vi "Save PNG File.vi"() -> (0 "ErrOut":errorcluster)   [LabVIEW 2017]
doc: "Use this template to build a VI to use as a subVI."
panel:
  out "ImageOut":T1(plugin-control)
  in  "ErrIn":errorcluster
  # "Input Parameters"
  # "Output Parameters"
  # "VI Description:\nThis VI is .."
  # ":: MVI Framework V1.0 ::\nAuthor:Gaoke Yang\nEmail: gaoke.yang@yahoo.com\nWeb: www.mvicontrol.com\nCopyright (C) , MVI Technologies All Rights Reserved"
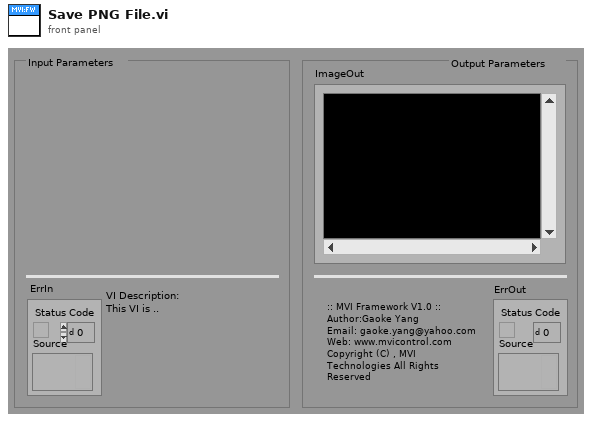
[diagram p1: front panel]
types:
  T1 = typedef "IMAQ Image.ctl" = refnum<image>
  T2 = typedef "Image Type" = u32
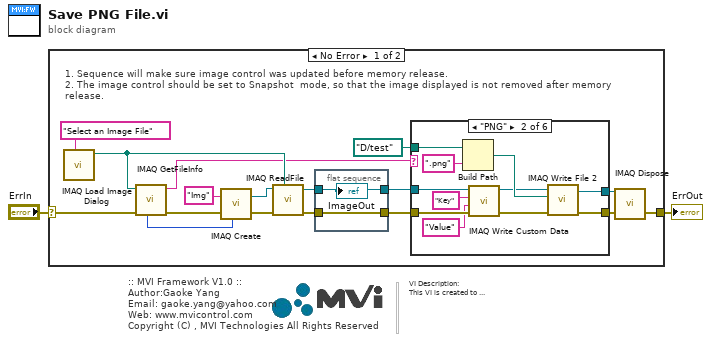
[diagram p0: block diagram]
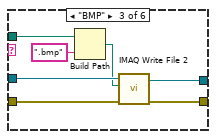
[diagram p3: hidden frame]
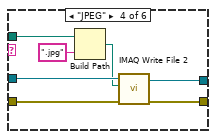
[diagram p4: hidden frame]
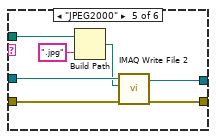
[diagram p5: hidden frame]
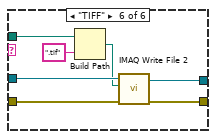
[diagram p6: hidden frame]
diagram:
  # "VI Description:\nThis VI is created to ..."
  # ":: MVI Framework V1.0 ::\nAuthor:Gaoke Yang\nEmail: gaoke.yang@yahoo.com\nWeb: www.mvicontrol.com\nCopyright (C) , MVI Technologies All Rights Reserved"
  n1 = case shown="No Error" "ErrIn" {
    selector: "ErrIn" -> [w14 w62]
    tunnel: [w13 w62] -> w2
    frame No Error {
      # "1. Sequence will make sure image control was updated before memory release.\n2. The image control should be set to Snapshot  mode, so that the image displayed is not removed after memory release."
      n2 = call "IMAQ Load Image Dialog"("Prompt"="Select an Image File" ("prompt")) -> ("Path"=w11:path)  [unwired: 8 in, 2 out]
      n3 = call "IMAQ GetFileInfo"("error in (no error)"=w14, "File Path"=w11) -> ("error out"=w15:errorcluster, "File Type"=w4:string, "Image Type"=w5:T2)  [unwired: 3 in, 4 out]
      n4 = call "IMAQ Create"("Image Name"="Img", "Image Type"=w5, "error in (no error)"=w15) -> ("New Image"=w18:T1, "error out"=w17:errorcluster)  [unwired: 2 in]
      n5 = call "IMAQ ReadFile"("File Path"=w11, "error in (no error)"=w17, "Image"=w18) -> ("error out"=w12:errorcluster, "Image Out"=w10:T1)  [unwired: 4 in, 3 out]
      n6 = flat-sequence {
        tunnel: w10 -> [w60]
        tunnel: w12 -> [w61]
        tunnel: [w61] -> w8
        tunnel: [w60] -> w3
        frame #0 {
          "ImageOut" <- w60
        }
      }
      n7 = case shown="\"PNG\"" w4 {
        tunnel: w3 -> [w21 w31 w38 w45 w52 w59]
        tunnel: [w21 w29 w36 w43 w50 w57] -> w9
        tunnel: w8 -> [w20 w30 w37 w44 w51 w58]
        tunnel: [w20 w28 w35 w42 w49 w56] -> w7
        tunnel: path "D:/test" ("File Path") -> [_ w26 w33 w40 w47 w54]
        frame "xxx", Default {
          # "unkown file type, do nothing"
        }
        frame "PNG" {
          n8 = Build Path(base path=w26, name or relative path=".png") -> (appended path=w27:path)
          n9 = call "IMAQ Write Custom Data"("Custom Data In"="Value", "Key"="Key", "Image"=w31) -> ("Image Out"=w24:T1)  [unwired: 7 in, 1 out]
          n10 = call-poly "IMAQ Write File 2"("error in (no error)"=w30, "File Path"=w27, "Image"=w24) -> ("error out"=w28:errorcluster, "Image Out (duplicate)"=w29:T1)  [unwired: 7 in]
        }
        frame "BMP" {
          n11 = Build Path(base path=w33, name or relative path=".bmp") -> (appended path=w34:path)
          n12 = call-poly "IMAQ Write File 2"("error in (no error)"=w37, "File Path"=w34, "Image"=w38) -> ("error out"=w35:errorcluster, "Image Out (duplicate)"=w36:T1)  [unwired: 7 in]
        }
        frame "JPEG" {
          n13 = Build Path(base path=w40, name or relative path=".jpg") -> (appended path=w41:path)
          n14 = call-poly "IMAQ Write File 2"("error in (no error)"=w44, "File Path"=w41, "Image"=w45) -> ("error out"=w42:errorcluster, "Image Out (duplicate)"=w43:T1)  [unwired: 7 in]
        }
        frame "JPEG2000" {
          n15 = Build Path(base path=w47, name or relative path=".jpg") -> (appended path=w48:path)
          n16 = call-poly "IMAQ Write File 2"("error in (no error)"=w51, "File Path"=w48, "Image"=w52) -> ("error out"=w49:errorcluster, "Image Out (duplicate)"=w50:T1)  [unwired: 7 in]
        }
        frame "TIFF" {
          n17 = Build Path(base path=w54, name or relative path=".tif") -> (appended path=w55:path)
          n18 = call-poly "IMAQ Write File 2"("error in (no error)"=w58, "File Path"=w55, "Image"=w59) -> ("error out"=w56:errorcluster, "Image Out (duplicate)"=w57:T1)  [unwired: 7 in]
        }
      }
      n19 = call "IMAQ Dispose"("Image"=w9, "error in (no error)"=w7) -> ("error out"=w13:errorcluster)  [unwired: 4 in]
    }
    frame Error {
    }
  }
  "ErrOut" <- w2
